vi "Emit_String.vi"(8 "Error In":errorcluster, 9 "Data":string, 10 "Signal Name":string, 11 "LQObject In":refnum<class "LQObject.lvclass">) -> (0 "Error Out":errorcluster, 3 "LQObject Out":refnum<class "LQObject.lvclass">)   [LabVIEW 2014, in "LQ Core.lvlib" / "LQObject.lvclass"]
uses:
  LQObject.lvclass
  LQIdentity/LQIdentity.lvclass/LQIdentity.ctl
  LQ Core.lvlib
  LQIdentity/LQIdentity.lvclass
panel:
  # "Copyright (c) 2016 Sze Howe Koh\n\nThis Source Code Form is subject to the terms of the Mozilla Public\nLicense, v. 2.0. If a copy of the MPL was not distributed with this\nfile, You can obtain one at http://mozilla.org/MPL/2.0/."
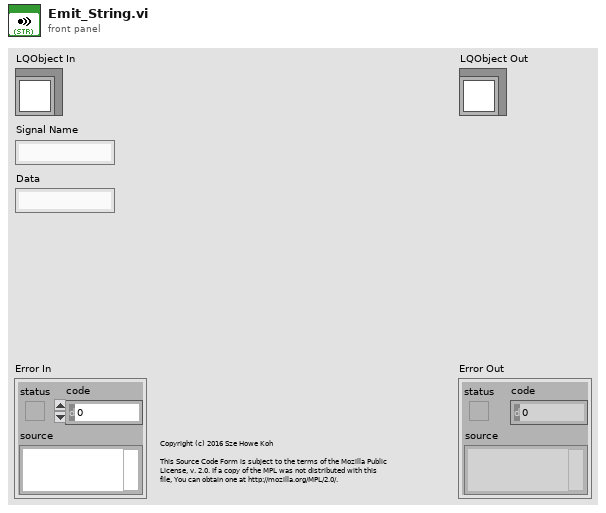
[diagram p1: front panel]
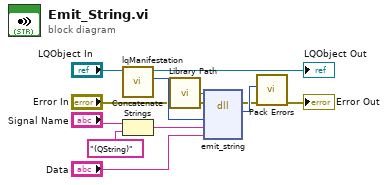
[diagram p0: block diagram]
diagram:
  n1 = call "lqManifestation.vi"("LQIdentity in"="LQObject In") -> ("Manifestation"=w5:u64, "LQIdentity out"=→"LQObject Out":refnum<class "LQObject.lvclass">)  [unwired: 9 in]
  n2 = Concatenate Strings("Signal Name", "(QString)") -> (w4:string)
  n3 = call "Library Path.vi"() -> ("Library Path"=w8:path)
  n4 = dll-call lib="?" fn="emit_string"(path in=w8, error in="Error In", "_instance"=w5, "normalizedSignal"=w4, "data"="Data") -> (error out=w9:errorcluster, "errorCode"=w10:i32)  [unwired: 4 in, 1 out]
  n5 = call "Pack Errors.vi"("Error In"=w9, "Error Code"=w10) -> ("Error Out"=→"Error Out":errorcluster)  [unwired: 9 in]
